vi "Post Substeps Waveform Generation Start Task.vi"(10 "Socket No":u16=1, 11 "Sequence Context In":refnum<k7>) -> (0 "error out":errorcluster, 3 "Report Text":string)   [LabVIEW 2023, in "LTT_TeststandSteptypes.lvlib"]
doc: "This VI Is Socket Number based AO Data Signal Write Through Q"
uses:
  LTT_TeststandSteptypes.lvlib
panel:
  in  "AOWrite":T1 {"Signal Name List"."Waveform Type" items=["Sine Wave", "Triangle Wave", "Square Wave", "Sawtooth Wave"]}
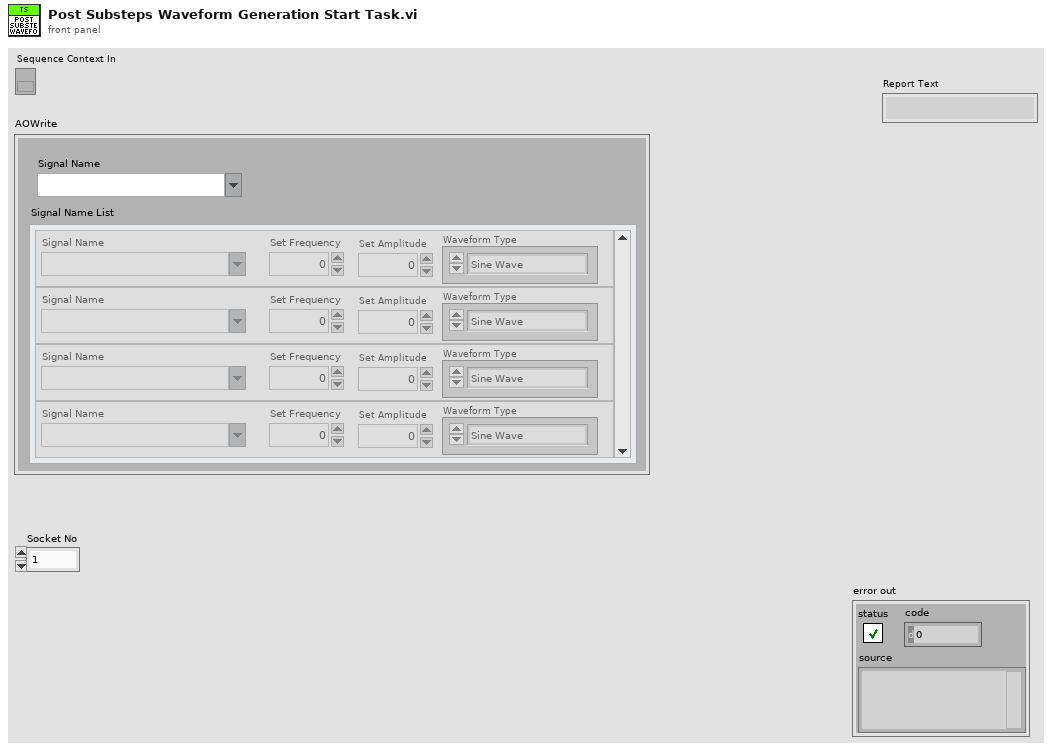
[diagram p1: front panel]
types:
  T1 = cluster{"Signal Name":string, "Signal Name List":cluster{"Signal Name":string, "Set Frequency":dbl, "Set Amplitude":dbl, "Waveform Type":u16}[]}
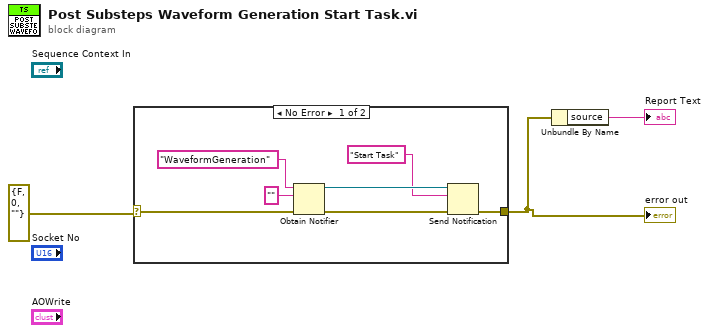
[diagram p0: block diagram]
diagram:
  n1 = case shown="No Error" errorcluster {"status"=FALSE, "code"=0, "source"=""} ("error in") {
    selector: errorcluster {"status"=FALSE, "code"=0, "source"=""} ("error in") -> [w4 w11]
    tunnel: [w5 w11] -> w1
    frame No Error {
      n2 = Obtain Notifier(name (unnamed)="WaveformGeneration", notification data type="", error in (no error)=w4) -> (notifier out=w10:refnum<notifier>, error out=w9:errorcluster)  [unwired: 1 in, 1 out]
      n3 = Send Notification(notification="Start Task", notifier=w10, error in (no error)=w9) -> (error out=w5:errorcluster)  [unwired: 1 out]
    }
    frame Error {
    }
  }
  "error out" <- w1
  n4 = Unbundle By Name(w1) -> ("source"=→"Report Text":string)
